vi "latt_grid.vi"(0 "pict in":picture, 1 "size":i32=40, 2 "nr lines":cluster{"x":i32, "y":i32}={"x"=7, "y"=15}, 3 "rotation":dbl[][](array[numeric]), 4 "Half sphere":bool, 5 "center":cluster{"x":i32, "y":i32}={"x"=44, "y"=44}) -> (6 "pict out":picture)   [LabVIEW 2017]
uses:
  <vilib>/Analysis/baseanly.llb/Real A x B.vi
  <vilib>/Analysis/NI_AALBase.lvlib
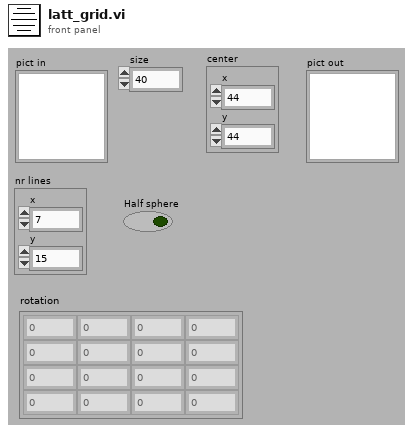
[diagram p1: front panel]
types:
  T1 = typedef "NI_Matrix.lvlib/RealMatrix.ctl" = dbl[][]
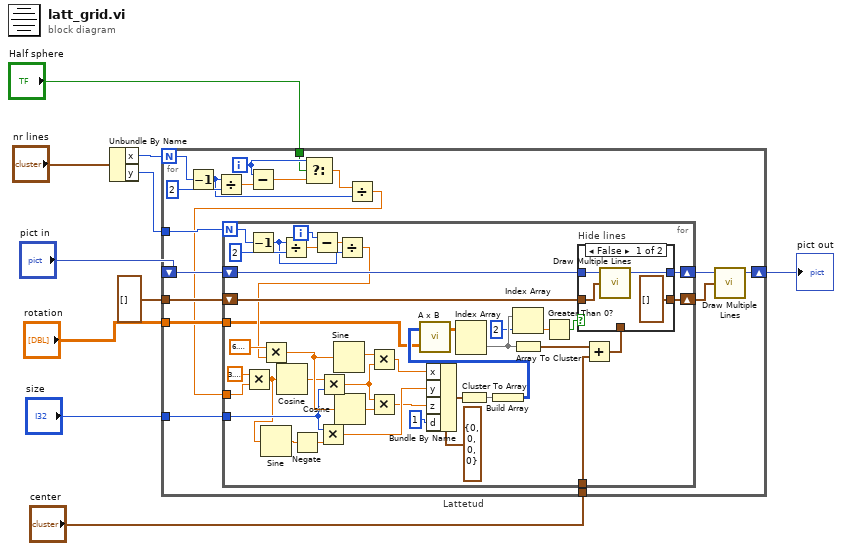
[diagram p0: block diagram]
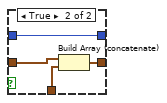
[diagram p2: hidden frame]
diagram:
  n1 = Unbundle By Name("nr lines") -> ("x"=w7:i32, "y"=w8:i32)
  n2 = for "Lattetud" {
    N: w7 -> [w25]
    tunnel: w8 -> [w28]
    shift-right: [w21] -> w4
    shift-left: "pict in" -> [w23]
    tunnel: "size" -> [w24]
    tunnel: cluster{"A x B[0]":dbl, "A x B[1]":dbl}[] [] -> [w19]
    tunnel: "rotation" -> [w17]
    tunnel: "center" -> [w15]
    tunnel: "Half sphere" -> [w11]
    i -> [w12]
    n3 = Decrement(x=w25) -> (x-1=w18:i32)
    n4 = Divide(x=w18, y=2) -> (x/y=w26:dbl)
    n5 = Subtract(x=w12, y=w26) -> (x-y=w13:dbl)
    n6 = Select(t=w12, s=w11, f=w13) -> (s? t:f=w14:dbl)
    n7 = Divide(x=w14, y=w18) -> (x/y=w16:dbl)
    n8 = for {
      N: w28 -> [w60]
      tunnel: w24 -> [w41]
      shift-right: [w54] -> w20
      shift-left: w19 -> [w53]
      shift-right: [w47] -> w22
      shift-left: w23 -> [w48]
      tunnel: w16 -> [w39]
      tunnel: w17 -> [w36]
      tunnel: w15 -> [w30]
      i -> [w65]
      n9 = Multiply(x=3.141592653589793, y=w39) -> (x*y=w35:dbl)
      n10 = Decrement(x=w60) -> (x-1=w55:i32)
      n11 = Sine(x=w35) -> (sin(x)=w31:dbl)
      n12 = Cosine(x=w35) -> (cos(x)=w57:dbl)
      n13 = Divide(x=w55, y=2) -> (x/y=w64:dbl)
      n14 = Negate(x=w31) -> (-x=w29:dbl)
      n15 = Subtract(x=w65, y=w64) -> (x-y=w58:dbl)
      n16 = Multiply(x=w41, y=w29) -> (x*y=w34:dbl)
      n17 = Multiply(x=w57, y=w41) -> (x*y=w56:dbl)
      n18 = Divide(x=w58, y=w55) -> (x/y=w40:dbl)
      n19 = Multiply(x=6.283185307179586, y=w40) -> (x*y=w62:dbl)
      n20 = Sine(x=w62) -> (sin(x)=w61:dbl)
      n21 = Cosine(x=w62) -> (cos(x)=w44:dbl)
      n22 = Multiply(x=w61, y=w56) -> (x*y=w59:dbl)
      n23 = Multiply(x=w56, y=w44) -> (x*y=w33:dbl)
      n24 = Bundle By Name(cluster=cluster{"x":i16, "y":i16, "z":i16, "d":i16} {"x"=0, "y"=0, "z"=0, "d"=0}, "x"=w59, "y"=w34, "z"=w33, "d"=i16 1) -> (w68:cluster{"x":i16, "y":i16, "z":i16, "d":i16})
      n25 = Cluster To Array(cluster=w68) -> (array=w67:i16[])
      n26 = Build Array(w67) -> (w38:i16[][])
      n27 = call-poly <vilib>:"A x B.vi"("B"=w36, "A"=w38) -> ("A x B"=w37:T1)  [unwired: 1 out]
      n28 = Index Array(array=w37) -> (element=w52:dbl[])  [unwired: 2 in]
      n29 = Index Array(array=w52, index=2) -> (element=w51:dbl)
      n30 = Array To Cluster(array=w52) -> (cluster=w46:cluster{"A x B[0]":dbl, "A x B[1]":dbl})
      n31 = Greater Than 0?(x=w51) -> (x > 0?=w50:bool)
      n32 = Add(x=w46, y=w30) -> (x+y=w45:cluster{dbl, dbl})
      n33 = case "Hide lines" shown="False" w50 {
        tunnel: [cluster{"A x B[0]":dbl, "A x B[1]":dbl}[] [] w76] -> w54
        tunnel: w53 -> [w69 w75]
        tunnel: w48 -> [w71 w74]
        tunnel: [w70 w74] -> w47
        tunnel: w45 -> [_ w73]
        frame False {
          n34 = call <vilib>:"Draw Multiple Lines.vi"("picture"=w71, "line endpoints"=w69) -> ("new picture"=w70:picture)  [unwired: 7 in]
        }
        frame True {
          n35 = Build Array (concatenate)(w75, w73) -> (w76:cluster{"A x B[0]":dbl, "A x B[1]":dbl}[])
        }
      }
    }
    n36 = call <vilib>:"Draw Multiple Lines.vi"("picture"=w22, "line endpoints"=w20) -> ("new picture"=w21:picture)  [unwired: 7 in]
  }
  "pict out" <- w4
